vi "svc_Peel String.vi"(10 "string":string="(EU)") -> (2 "peeled string":string)   [LabVIEW 2017]
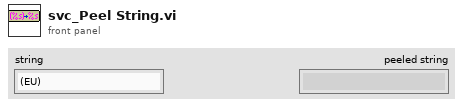
[diagram p1: front panel]
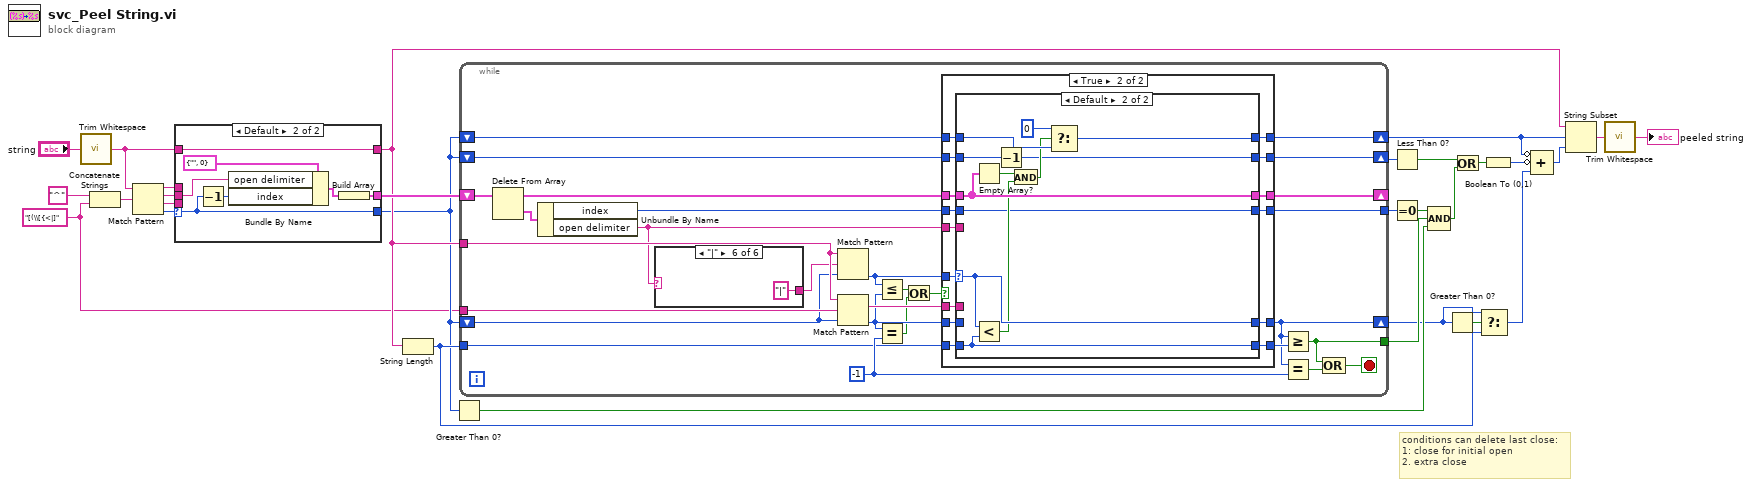
[diagram p0: block diagram]
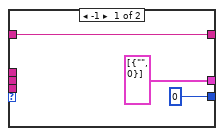
[diagram p2: hidden frame]
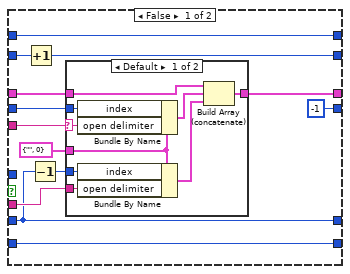
[diagram p3: hidden frame]
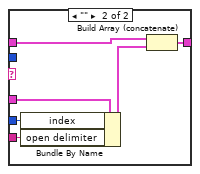
[diagram p4: hidden frame]
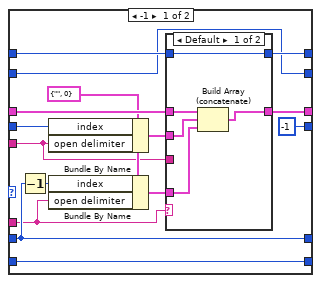
[diagram p5: hidden frame]
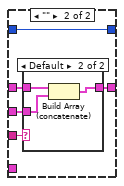
[diagram p6: hidden frame]
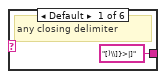
[diagram p8: hidden frame]
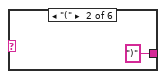
[diagram p9: hidden frame]
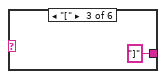
[diagram p10: hidden frame]
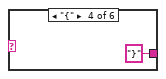
[diagram p11: hidden frame]
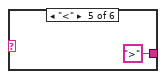
[diagram p12: hidden frame]
diagram:
  w3 = "[(\\[{<|]" ("regular expression")
  # "conditions can delete last close:\n1: close for initial open\n2. extra close"
  n1 = call <vilib>:"Trim Whitespace.vi"("string"="string") -> ("trimmed string"=w23:string)  [unwired: 1 in]
  n2 = Concatenate Strings("^" ("regular expression"), w3) -> (w1:string)
  n3 = Match Pattern(string=w23, regular expression=w1) -> (before substring=w25:string, match substring=w22:string, after substring=w24:string, offset past match=w27:i32)  [unwired: 1 in]
  n4 = case shown="Default" w27 {
    selector: w27 -> [_ w36]
    tunnel: w22 -> [_ w37]
    tunnel: [cluster{"open delimiter":string, "index":i32}[] [{"open delimiter"="", "index"=0}] w39] -> w26
    tunnel: w25 -> [_ _]
    tunnel: w24 -> [_ _]
    tunnel: [w32 w38] -> w15
    tunnel: w23 -> [w32 w38]
    tunnel: [0 ("offset past match") w36] -> w5
    frame -1 {
    }
    frame Default {
      n5 = Decrement(x=w36) -> (x-1=w35:i32)
      n6 = Bundle By Name(cluster=cluster{"open delimiter":string, "index":i32} {"open delimiter"="", "index"=0}, "open delimiter"=w37, "index"=w35) -> (w33:cluster{"open delimiter":string, "index":i32})
      n7 = Build Array(w33) -> (w39:cluster{"open delimiter":string, "index":i32}[])
    }
  }
  n8 = String Length(string=w15) -> (length=w17:i32)
  n9 = Greater Than 0?(x=w5) -> (x > 0?=w7:bool)
  n10 = while {
    tunnel: w15 -> [w65]
    shift-right: [w49] -> w4
    shift-left: w5 -> [w43]
    shift-right: [w46] -> _
    shift-left: w26 -> [w67]
    tunnel: w17 -> [w51]
    tunnel: w3 -> [w66]
    tunnel: [w54] -> w11
    shift-right: [w52] -> w14
    shift-left: w5 -> [w53]
    shift-right: [w45] -> w13
    shift-left: w5 -> [w47]
    tunnel: [w40] -> w6
    stop <- w60 stop-if-true
    w55 = -1 ("y")
    n11 = Delete From Array(array=w67) -> (deleted portion=w44:cluster{"open delimiter":string, "index":i32}, array with subset deleted=w63:cluster{"open delimiter":string, "index":i32}[])  [unwired: 2 in]
    n12 = Unbundle By Name(w44) -> ("index"=w41:i32, "open delimiter"=w42:string)
    n13 = case shown="\"|\"" w42 {
      tunnel: ["[)\\]}>|]" ")" "]" "}" ">" "|"] -> w61
      frame Default {
        # "any closing delimiter"
      }
      frame "(" {
      }
      frame "[" {
      }
      frame "{" {
      }
      frame "<" {
      }
      frame "|" {
      }
    }
    n14 = Match Pattern(string=w65, regular expression=w61, offset (0)=w43) -> (offset past match=w64:i32)  [unwired: 3 out]
    n15 = Match Pattern(string=w65, regular expression=w66, offset (0)=w43) -> (match substring=w62:string, offset past match=w59:i32)  [unwired: 2 out]
    n16 = Less Or Equal?(x=w64, y=w59) -> (x <= y?=w58:bool)
    n17 = Equal?(x=w59, y=w55) -> (x = y?=w57:bool)
    n18 = Or(x=w58, y=w57) -> (x .or. y?=w56:bool)
    n19 = case shown="True" w56 {
      tunnel: w64 -> [_ w110]
      tunnel: w63 -> [w80 w107]
      tunnel: [w78 w105] -> w46
      tunnel: w62 -> [w79 w106]
      tunnel: w42 -> [w77 w104]
      tunnel: [w71 w108] -> w49
      tunnel: w59 -> [w71 w109]
      tunnel: w53 -> [w76 w103]
      tunnel: [w76 w102] -> w52
      tunnel: w51 -> [w75 w101]
      tunnel: [w75 w100] -> w50
      tunnel: [w73 w99] -> w45
      tunnel: w47 -> [w74 w98]
      tunnel: w41 -> [w72 w97]
      tunnel: [-1 ("index") w96] -> w40
      frame False {
        n20 = Increment(x=w74) -> (x+1=w73:i32)
        n21 = Decrement(x=w71) -> (x-1=w70:i32)
        n22 = case shown="Default" w77 {
          selector: w77 -> [w86 _]
          tunnel: w80 -> [w89 w95]
          tunnel: w79 -> [w84 w91]
          tunnel: [w88 w94] -> w78
          tunnel: w72 -> [w87 _]
          tunnel: w70 -> [w82 w93]
          tunnel: cluster{"open delimiter":string, "index":i32} {"open delimiter"="", "index"=0} ("cluster") -> [w81 w92]
          frame Default {
            n23 = Bundle By Name(cluster=w81, "index"=w87, "open delimiter"=w86) -> (w85:cluster{"open delimiter":string, "index":i32})
            n24 = Bundle By Name(cluster=w81, "index"=w82, "open delimiter"=w84) -> (w83:cluster{"open delimiter":string, "index":i32})
            n25 = Build Array (concatenate)(w89, w85, w83) -> (w88:cluster{"open delimiter":string, "index":i32}[])
          }
          frame "" {
            n26 = Bundle By Name(cluster=w92, "index"=w93, "open delimiter"=w91) -> (w90:cluster{"open delimiter":string, "index":i32})
            n27 = Build Array (concatenate)(w95, w90) -> (w94:cluster{"open delimiter":string, "index":i32}[])
          }
        }
      }
      frame True {
        n28 = case shown="Default" w110 {
          selector: w110 -> [_ w146]
          tunnel: w109 -> [w117 _]
          tunnel: [w117 w146] -> w108
          tunnel: w107 -> [w125 w151]
          tunnel: w106 -> [w115 _]
          tunnel: [w124 w151] -> w105
          tunnel: w104 -> [w114 _]
          tunnel: w103 -> [w122 w150]
          tunnel: [w123 w148] -> w102
          tunnel: w101 -> [w121 w145]
          tunnel: [w121 w145] -> w100
          tunnel: [w111 w141] -> w99
          tunnel: w98 -> [w111 w142]
          tunnel: w97 -> [w120 w140]
          tunnel: [-1 ("index") w140] -> w96
          frame -1 {
            w118 = cluster{"open delimiter":string, "index":i32} {"open delimiter"="", "index"=0} ("cluster")
            n29 = Decrement(x=w117) -> (x-1=w116:i32)
            n30 = Bundle By Name(cluster=w118, "index"=w120, "open delimiter"=w114) -> (w119:cluster{"open delimiter":string, "index":i32})
            n31 = Bundle By Name(cluster=w118, "index"=w116, "open delimiter"=w115) -> (w113:cluster{"open delimiter":string, "index":i32})
            n32 = case shown="Default" w115 {
              tunnel: w125 -> [w130 w135]
              tunnel: [w129 w134] -> w124
              tunnel: w119 -> [w128 w131]
              tunnel: [w127 w133] -> w123
              tunnel: w122 -> [w127 w133]
              tunnel: w114 -> [_ w132]
              tunnel: w113 -> [w126 _]
              frame Default {
                n33 = Build Array (concatenate)(w130, w128, w126) -> (w129:cluster{"open delimiter":string, "index":i32}[])
              }
              frame "" {
                n34 = case shown="Default" w132 {
                  tunnel: w135 -> [w136 w139]
                  tunnel: [w136 w138] -> w134
                  tunnel: w131 -> [_ w137]
                  frame "" {
                  }
                  frame Default {
                    n35 = Build Array (concatenate)(w139, w137) -> (w138:cluster{"open delimiter":string, "index":i32}[])
                  }
                }
              }
            }
          }
          frame Default {
            n36 = Empty Array?(array=w151) -> (empty?=w144:bool)
            n37 = Less?(x=w146, y=w145) -> (x < y?=w143:bool)
            n38 = Decrement(x=w142) -> (x-1=w141:i32)
            n39 = And(x=w144, y=w143) -> (x .and. y?=w147:bool)
            n40 = Select(t=0, s=w147, f=w150) -> (s? t:f=w148:i32)
          }
        }
      }
    }
    n41 = Greater Or Equal?(x=w49, y=w50) -> (x >= y?=w54:bool)
    n42 = Equal?(x=w49, y=w55) -> (x = y?=w48:bool)
    n43 = Compound Arithmetic op=OR(w54, w48) -> (w60:bool)
  }
  n44 = Less Than 0?(x=w13) -> (x < 0?=w9:bool)
  n45 = Equal To 0?(x=w6) -> (x = 0?=w12:bool)
  n46 = Compound Arithmetic op=AND(w12, w11, w7) -> (w10:bool)
  n47 = Greater Than 0?(x=w4) -> (x > 0?=w18:bool)
  n48 = Or(x=w9, y=w10) -> (x .or. y?=w8:bool)
  n49 = Select(t=w4, s=w18, f=w17) -> (s? t:f=w19:i32)
  n50 = Boolean To (0,1)(Boolean=w8) -> (0, 1=w16:i16)
  n51 = Compound Arithmetic op=ADD(invert w14, invert w16, w19) -> (w21:i32)
  n52 = String Subset(string=w15, offset (0)=w14, length (rest)=w21) -> (substring=w20:string)
  n53 = call <vilib>:"Trim Whitespace.vi"("string"=w20) -> ("trimmed string"=→"peeled string":string)  [unwired: 1 in]
